vi "tb_06-ni.vi"(0 "Etude":T2, 1 "Aff ?":bool, 5 "VS":T4, 7 "ent-2D":string[][](array[string]), 9 "do-2D":string[][](array[string]), 11 "tb in ?":bool[](array[boolean])) -> (4 "Etude":T2, 6 "VS":T4, 8 "ent-2D":T1[][](array[typedef]), 10 "do-2D":string[][](array[string]), 12 "Xc":string[](array[string]), 13 "Xc-ent":T1, 14 "Xc-lib":T1, 15 "tb in ?":bool[](array[boolean]))   [LabVIEW 2010, in "lv_04.lvlib"]
uses:
  lv_04/lv_04.lvlib
  lv_04/commandes/cX.ctl
  lv_04/commandes/cSTA_varid.ctl
  lv_04/commandes/c_TDMS_ch_variable.ctl
  lv_04/commandes/c_TDMS_ch_donnees.ctl
  lv_04/commandes/c0-var-n.ctl
  lv_04/commandes/cSTA_num_do_cr.ctl
  lv_04/commandes/c02-do-num.ctl
  lv_04/commandes/c04-stat-num.ctl
  lv_04/commandes/cSTA_txt_do_cr.ctl
  lv_04/commandes/c02-do-txt.ctl
  lv_04/commandes/c04-stat-txt.ctl
  lv_04/commandes/cSTA_dist.ctl
  lv_04/commandes/c03-dist-S.ctl
  lv_04/commandes/c0-dist-xy.ctl
  lv_04/commandes/c03-dist-T.ctl
  lv_04/commandes/c03-dist-SPC.ctl
  lv_04/commandes/c_etude.ctl
  lv_02/p_5E_ch_loi.ctl
  lv_01/type format.ctl
  lv_01/lv_01.lvlib
  lv_02/lv_02.lvlib
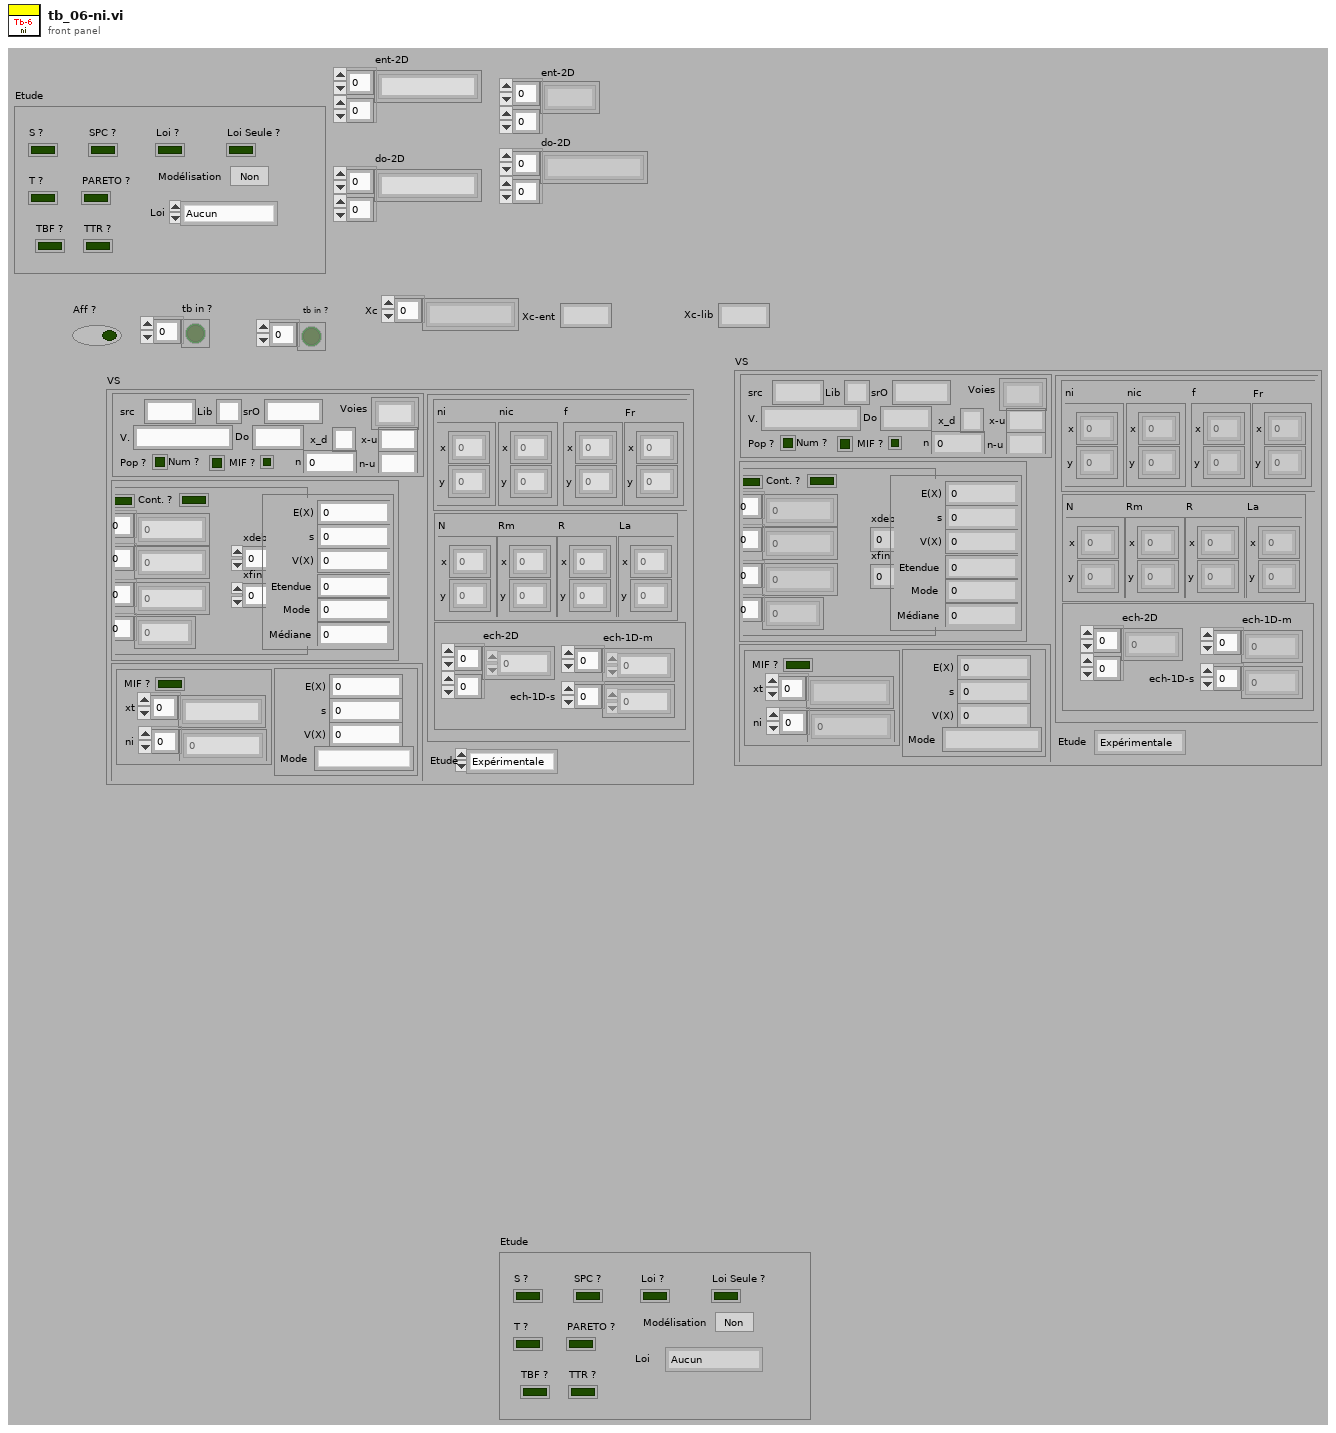
[diagram p1: front panel]
types:
  T1 = typedef "lv_04.lvlib/c_TDMS_ch_donnees.ctl" = string
  T2 = typedef "lv_04.lvlib/c_etude.ctl" = cluster{"T ?":bool, "S ?":bool, "SPC ?":bool, "PARETO ?":bool, "TBF ?":bool, "TTR ?":bool, "Loi ?":bool, "Loi Seule ?":bool, "Modélisation":bool, "Loi":T3}
  T3 = typedef "lv_02.lvlib/p_5E_ch_loi.ctl" = enum16{"Aucun", "Normale", "Aucun2", "Aucun3", "Binômial", "Poisson", "Exponentiel", "Weibull", "Rang médian"}
  T4 = typedef "lv_04.lvlib/cX.ctl" = cluster{"src":T5, "num":T8, "txt":T11, "dist":T14, "Etude":enum16{"Expérimentale", "Modèle"}}
  T5 = typedef "lv_04.lvlib/cSTA_varid.ctl" = cluster{"src":string, "Lib":string, "srO":string, "V.":T6, "Voies":string[], "Do":T1, "n":T7, "Num ?":bool, "Pop ?":bool, "x_d":string, "x-u":string, "n-u":string, "MIF ?":bool}
  T6 = typedef "lv_04.lvlib/c_TDMS_ch_variable.ctl" = string
  T7 = typedef "lv_04.lvlib/c0-var-n.ctl" = i32
  T8 = typedef "lv_04.lvlib/cSTA_num_do_cr.ctl" = cluster{"do":T9, "sta":T10}
  T9 = typedef "lv_04.lvlib/c02-do-num.ctl" = cluster{"MIF ?":bool, "Cont. ?":bool, "xi":dbl[], "xic":dbl[], "ni":u32[], "dx":dbl[], "xdeb":dbl, "xfin":dbl}
  T10 = typedef "lv_04.lvlib/c04-stat-num.ctl" = cluster{"E(X)":dbl, "s":dbl, "V(X) ":dbl, "Etendue":dbl, "Mode":dbl, "Médiane":dbl}
  T11 = typedef "lv_04.lvlib/cSTA_txt_do_cr.ctl" = cluster{"do":T12, "sta":T13}
  T12 = typedef "lv_04.lvlib/c02-do-txt.ctl" = cluster{"xt":string[], "ni":dbl[], "MIF ?":bool}
  T13 = typedef "lv_04.lvlib/c04-stat-txt.ctl" = cluster{"E(X)":dbl, "s":dbl, "V(X) ":dbl, "Mode":string}
  T14 = typedef "lv_04.lvlib/cSTA_dist.ctl" = cluster{"S":T15, "T":T17, "spc":T18}
  T15 = typedef "lv_04.lvlib/c03-dist-S.ctl" = cluster{"nic":T16, "f":T16, "Fr":T16, "ni":T16}
  T16 = typedef "lv_04.lvlib/c0-dist-xy.ctl" = cluster{"x":dbl[], "y":dbl[]}
  T17 = typedef "lv_04.lvlib/c03-dist-T.ctl" = cluster{"N":T16, "Rm":T16, "R":T16, "La":T16}
  T18 = typedef "lv_04.lvlib/c03-dist-SPC.ctl" = cluster{"ech-2D":dbl[][], "ech-1D-m":dbl[], "ech-1D-s":dbl[]}
  T19 = typedef "lv_01.lvlib/type format.ctl" = enum16{"X (dbl)", "P (Proba)", "N (entier)", "S (Scient.)"}
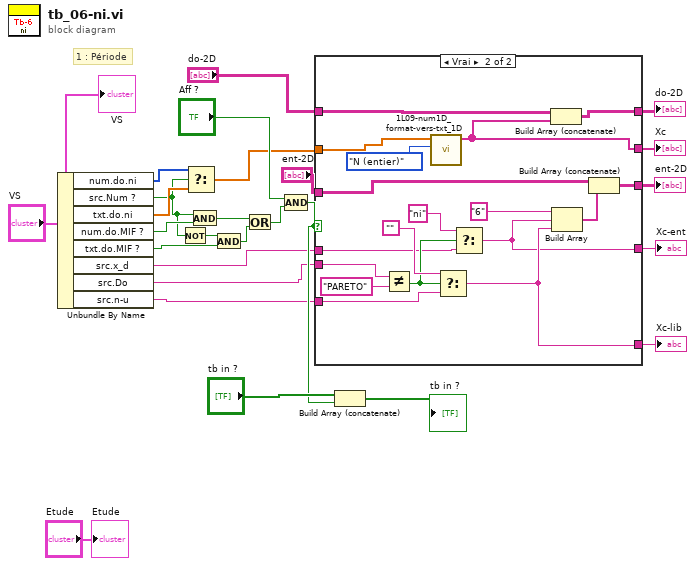
[diagram p0: block diagram]
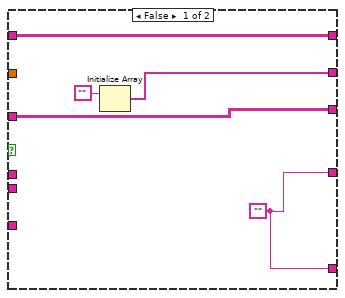
[diagram p2: hidden frame]
diagram:
  # "1 : Période"
  n1 = Unbundle By Name("VS") -> ("num.do.ni"=w13:u32[], "src.Num ?"=w9:bool, "txt.do.ni"=w12:dbl[], "num.do.MIF ?"=w10:bool, "txt.do.MIF ?"=w7:bool, "src.x_d"=w2:string, "src.Do"=w1:T1, "src.n-u"=w3:string)
  n2 = Not(x=w9) -> (.not. x?=w8:bool)
  n3 = Select(t=w13, s=w9, f=w12) -> (s? t:f=w11:dbl[])
  n4 = And(x=w9, y=w10) -> (x .and. y?=w5:bool)
  n5 = And(x=w8, y=w7) -> (x .and. y?=w6:bool)
  n6 = Or(x=w5, y=w6) -> (x .or. y?=w4:bool)
  n7 = Compound Arithmetic op=AND("Aff ?", w4) -> (w15:bool)
  n8 = case shown="Vrai" w15 {
    tunnel: w11 -> [_ w43]
    tunnel: [w31 w41] -> w24
    tunnel: w1 -> [_ w33]
    tunnel: "do-2D" -> [w29 w49]
    tunnel: [w29 w48] -> w22
    tunnel: "ent-2D" -> [w28 w47]
    tunnel: [w28 w45] -> w20
    tunnel: [w27 w32] -> w19
    tunnel: [w27 w37] -> w18
    tunnel: w3 -> [_ w38]
    tunnel: w2 -> [_ w34]
    frame False {
      w27 = ""
      n9 = Initialize Array("") -> (w31:string[])  [unwired: 1 in]
    }
    frame True {
      n10 = Not Equal?(x=w33, y=T1 "PARETO") -> (x != y?=w36:bool)
      n11 = call "1L09-num1D_format-vers-txt_1D.vi"("type"=type_format."N (entier)", "1D( num)"=w43) -> ("1D (ch)"=w41:string[])  [unwired: 7 in]
      n12 = Select(t="", s=w36, f=w38) -> (s? t:f=w37:string)
      n13 = Select(t="ni", s=w36, f=w34) -> (s? t:f=w32:string)
      n14 = Build Array (concatenate)(w49, w41) -> (w48:string[][])
      n15 = Build Array("6", w32, w37) -> (w46:string[])
      n16 = Build Array (concatenate)(w47, w46) -> (w45:string[][])
    }
  }
  "Xc" <- w24
  "Xc-ent" <- w19
  "Xc-lib" <- w18
  "ent-2D" <- w20
  "do-2D" <- w22
  n17 = Build Array (concatenate)("tb in ?", w15) -> (→"tb in ?":bool[])
  "VS" <- "VS"
  "Etude" <- "Etude"
